vi "Read Voltage.vi"(8 "error in":errorcluster, 11 "Modbus instance in":refnum<class "Modbus API.lvclass">) -> (0 "error out":errorcluster, 2 "Voltage Read":dbl, 3 "Modbus instance out":refnum<class "Modbus API.lvclass">)   [LabVIEW 2025, in "Hanmatek HM310T.lvlib"]
uses:
  <vilib>/NI/Modbus Library/API/Modbus API.lvclass
  <instrlib>/Hanmatek HM310T/Hanmatek HM310T.lvlib
  3c5996ca-f78e-4e41-a5a2-f34556adb45b.vi
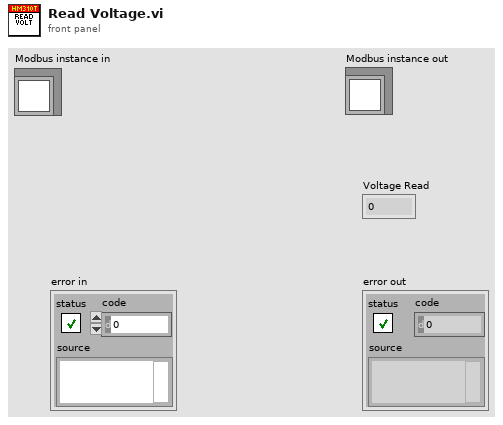
[diagram p1: front panel]
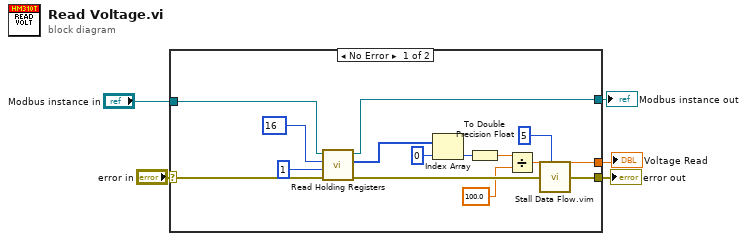
[diagram p0: block diagram]
diagram:
  n1 = case shown="No Error" "error in" {
    selector: "error in" -> [w18 w21]
    tunnel: [w7 w21] -> w4
    tunnel: [w16 w20] -> w2
    tunnel: [w10 _] -> w3
    tunnel: "Modbus instance in" -> [w9 w20]
    frame No Error {
      n2 = call-dynamic "Read Holding Registers.vi"("error in"=w18, "number of inputs"=u16 1, "starting address"=u16 16 ("Quantity of words (1)"), "Modbus instance in"=w9) -> ("error out"=w17:errorcluster, "register values"=w15:u16[], "Modbus instance out"=w16:refnum<class "Modbus API.lvclass">)  [unwired: 5 in]
      n3 = Index Array(array=w15, index=0) -> (element=w13:u16)
      n4 = To Double Precision Float(number=w13) -> (double precision float=w11:dbl)
      n5 = Divide(x=w11, y=100.0) -> (x/y=w10:dbl)
      n6 = call "Stall Data Flow.vim"("value in"=w17, "milliseconds to wait"=u32 5) -> ("value out"=w7:errorcluster)  [unwired: 1 out]
    }
    frame Error {
    }
  }
  "error out" <- w4
  "Voltage Read" <- w3
  "Modbus instance out" <- w2
